vi "Destroy Timer Handler.vi"(8 "error in (no error)":errorcluster, 11 "Timer Handler":T1) -> (0 "error out":errorcluster)   [LabVIEW 2024]
doc: "Destroys timer handlers."
uses:
  Timer Handler.ctl
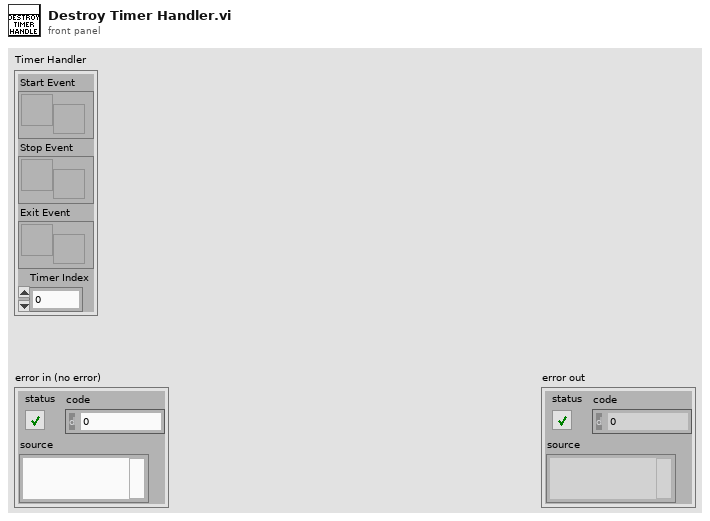
[diagram p1: front panel]
types:
  T1 = typedef "Timer Handler.ctl" = cluster{"Start Event":refnum<user-event>, "Stop Event":refnum<user-event>, "Exit Event":refnum<user-event>, "Timer Index":u32}
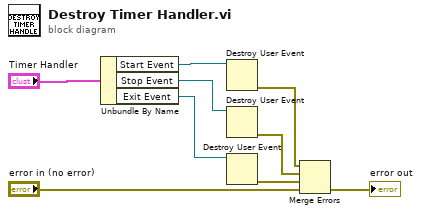
[diagram p0: block diagram]
diagram:
  n1 = Unbundle By Name("Timer Handler") -> ("Start Event"=w6:refnum<user-event>, "Stop Event"=w5:refnum<user-event>, "Exit Event"=w4:refnum<user-event>)
  n2 = Destroy User Event(user event=w6) -> (error out=w3:errorcluster)  [unwired: 1 in]
  n3 = Destroy User Event(user event=w5) -> (error out=w2:errorcluster)  [unwired: 1 in]
  n4 = Destroy User Event(user event=w4) -> (error out=w1:errorcluster)  [unwired: 1 in]
  n5 = Merge Errors(w3, w2, w1, "error in (no error)") -> (→"error out":errorcluster)
